vi "id.To JSON Tree.vi"(8 "error in (no error)":errorcluster, 11 "id in":refnum<class "id.lvclass">) -> (0 "error out":errorcluster, 2 "JSON Value out":refnum<class "JSON Value.lvclass">, 3 "id out":refnum<class "id.lvclass">)   [LabVIEW 2016, in "id.lvclass"]
uses:
  id.lvclass
  <vilib>/NI/JSON Support for LabVIEW/JSON Value/JSON Value.lvclass
  id.lvclass/id.ctl
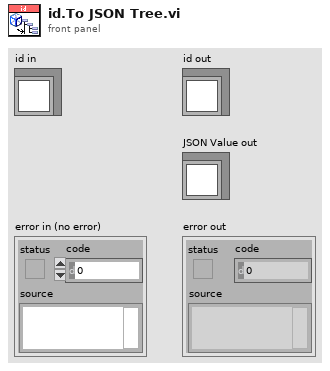
[diagram p1: front panel]
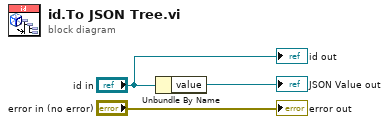
[diagram p0: block diagram]
diagram:
  n1 = Unbundle By Name("id in") -> ("value"=→"JSON Value out":refnum<class "JSON Value.lvclass">)
  "error out" <- "error in (no error)"
  "id out" <- "id in"
